vi "Preview Appended Waveform List.vi"(8 "error in (no error)":errorcluster, 10 "Trim and Resample Settings":cluster{"Duration":dbl, "Sample Rate":dbl}={"Duration"=0.002, "Sample Rate"=0.0} {"Sample Rate" format="%#_6pHz"; "Duration" format="%#_6ps"}, 11 "Canvas Wfm Array In":waveform(dbl)[](array[waveform])) -> (0 "error out":errorcluster, 2 "Final Waveform":waveform(dbl), 3 "Canvas Wfm Array Out":waveform(dbl)[](array[waveform]))   [LabVIEW 2025, in "TDMS Waveform Creator UI.lvlib"]
uses:
  TDMS Waveform Creator UI.lvlib
  <vilib>/Waveform/WDTOps.llb/WDT Append Waveforms DBL.vi
  <vilib>/Waveform/WDTOps.llb/WDT Waveform Duration DBL.vi
  <vilib>/Waveform/WDTOps.llb/WDT Get Waveform Subset DBL.vi
  <vilib>/measure/maresamp.llb/Resample Waveform (single shot).vi
  <vilib>/measure/NI_MAPro.lvlib
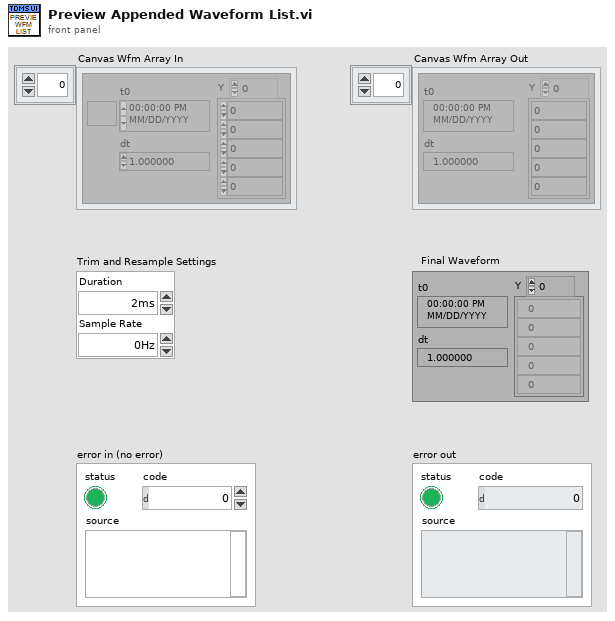
[diagram p1: front panel]
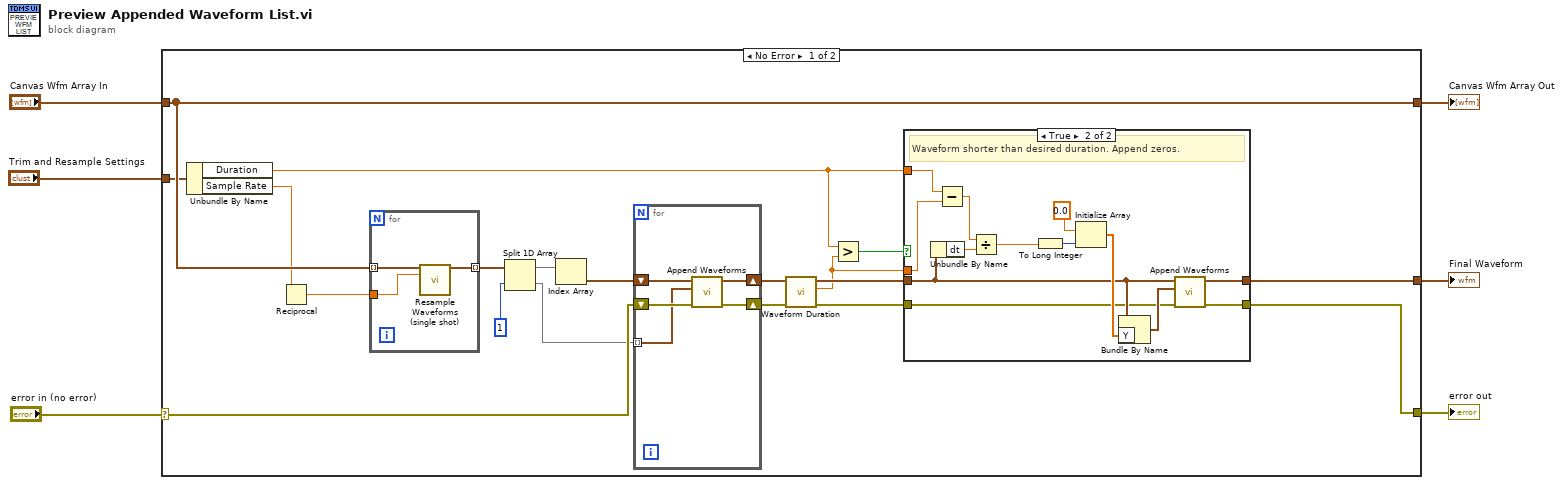
[diagram p0: block diagram]
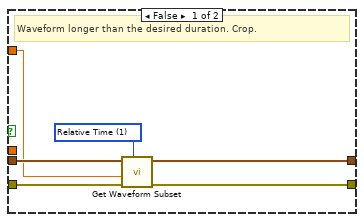
[diagram p2: hidden frame]
diagram:
  n1 = case shown="No Error" "error in (no error)" {
    selector: "error in (no error)" -> [w25 w54]
    tunnel: "Canvas Wfm Array In" -> [w24 w53]
    tunnel: [w24 w53] -> w4
    tunnel: "Trim and Resample Settings" -> [w23 _]
    tunnel: [w15 _] -> w2
    tunnel: [w14 w54] -> w1
    frame No Error {
      n2 = Unbundle By Name(w23) -> ("Duration"=w9:dbl, "Sample Rate"=w22:dbl)
      n3 = Reciprocal(x=w22) -> (1/x=w21:dbl)
      n4 = for {
        tunnel: w24 -> [w52] mode=indexing
        tunnel: w21 -> [w51]
        tunnel: [w50] -> w20 mode=indexing
        n5 = call-poly <vilib>:"Resample Waveforms (single shot).vi"("waveform in"=w52, "dt"=w51) -> ("resampled waveform out"=w50:waveform(dbl))  [unwired: 10 in, 3 out]
      }
      n6 = Split 1D Array(array=w20, index=1) -> (first subarray=w19:waveform(dbl)[], second subarray=w17:waveform(dbl)[])
      n7 = Index Array(array=w19) -> (element=w18:waveform(dbl))  [unwired: 1 in]
      n8 = for {
        shift-right: [w48] -> w11
        shift-left: w18 -> [w49]
        tunnel: w17 -> [w45] mode=indexing
        shift-right: [w46] -> w16
        shift-left: w25 -> [w47]
        n9 = call-poly <vilib>:"Append Waveforms.vi"("error in (no error)"=w47, "waveform B"=w45, "waveform A"=w49) -> ("error out"=w46:errorcluster, "waveform out"=w48:waveform(dbl))  [unwired: 7 in]
      }
      n10 = call-poly <vilib>:"Waveform Duration.vi"("error in (no error)"=w16, "waveform in"=w11) -> ("error out"=w12:errorcluster, "duration"=w8:dbl, "waveform out"=w10:waveform(dbl))  [unwired: 7 in]
      n11 = Greater?(x=w9, y=w8) -> (0:w7:bool)
      n12 = case shown="True" w7 {
        tunnel: [w31 w35] -> w15
        tunnel: [w30 w33] -> w14
        tunnel: w12 -> [w29 w34]
        tunnel: w10 -> [w28 w36]
        tunnel: w9 -> [w27 w43]
        tunnel: w8 -> [_ w44]
        frame False {
          w26 = u16 1 items=["Samples", "Relative Time"] ("start/duration format")
          # "Waveform longer than the desired duration. Crop."
          n13 = call-poly <vilib>:"Get Waveform Subset.vi"("start/duration format"=w26, "error in (no error)"=w29, "duration"=w27, "waveform in"=w28) -> ("error out"=w30:errorcluster, "waveform out"=w31:waveform(dbl))  [unwired: 2 in, 2 out]
        }
        frame True {
          # "Waveform shorter than desired duration. Append zeros."
          n14 = Unbundle By Name(w36) -> ("dt"=w41:dbl)
          n15 = Subtract(x=w43, y=w44) -> (x-y=w42:dbl)
          n16 = Divide(x=w42, y=w41) -> (x/y=w32:dbl)
          n17 = To Long Integer(number=w32) -> (32bit integer=w40:i32)
          n18 = Initialize Array(0.0 ("element"), w40) -> (w38:dbl[])
          n19 = Bundle By Name(cluster=w36, "Y"=w38) -> (w37:waveform(dbl))
          n20 = call-poly <vilib>:"Append Waveforms.vi"("error in (no error)"=w34, "waveform B"=w37, "waveform A"=w36) -> ("error out"=w33:errorcluster, "waveform out"=w35:waveform(dbl))  [unwired: 7 in]
        }
      }
    }
    frame Error {
    }
  }
  "error out" <- w1
  "Canvas Wfm Array Out" <- w4
  "Final Waveform" <- w2
